vi "read_attributes.vi"(8 "error in (no error)":errorcluster, 11 "KernelRidge in":refnum<class "KernelRidge.lvclass">) -> (0 "error out":errorcluster, 2 "attributes":T1, 3 "KernelRidge out":refnum<class "KernelRidge.lvclass">)   [LabVIEW 2020, in "KernelRidge.lvclass"]
uses:
  KernelRidge.lvclass
  Controls/kernel_ridge_attributes.ctl
  KernelRidge.lvclass/KernelRidge.ctl
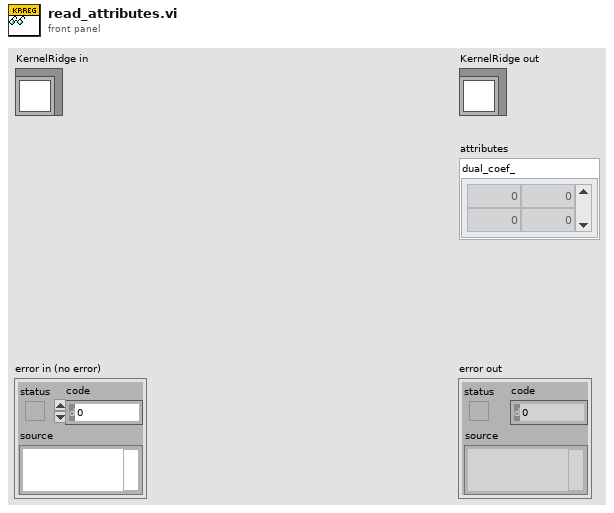
[diagram p1: front panel]
types:
  T1 = typedef "kernel_ridge_attributes.ctl" = cluster{"dual_coef_":dbl[][]}
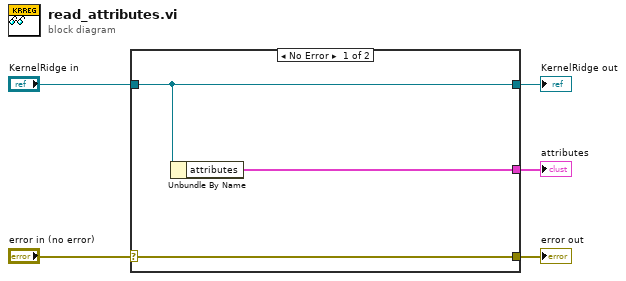
[diagram p0: block diagram]
diagram:
  n1 = case shown="No Error" "error in (no error)" {
    selector: "error in (no error)" -> [w8 w9]
    tunnel: [w8 w9] -> w4
    tunnel: [w7 w10] -> w2
    tunnel: "KernelRidge in" -> [w7 w10]
    tunnel: [w6 _] -> w1
    frame No Error {
      n2 = Unbundle By Name(w7) -> ("attributes"=w6:T1)
    }
    frame Error {
    }
  }
  "error out" <- w4
  "KernelRidge out" <- w2
  "attributes" <- w1
